vi "non_linear_fitting_multiple.vi"(11 "Graph array":cluster{"output":dbl[], "output":dbl[]}[](array[cluster])=[{"output"=array[10000 elements], "output"=array[10000 elements]}]) -> (0 "error out":errorcluster)   [LabVIEW 2025]
panel:
  in  "Old Fitting functions":string="standard streched expnental + power decay\n: (a0+a1*x^(a2)*exp(-(x/a3)^a4)\nstreched exponential with modified constants for x=0,limitless\n:(a0-a1)*exp(-(x/a2)^a3)+a1"
  out "Numeric":i32
  in  "fitting param col.":i32
  out "fitting parameter plot":cluster{dbl[], dbl[]}(graph)
  out "best fit parameter":dbl[](array[numeric])
  in  "Fitting Function":string="(a0-a1)*exp(-(x/a2)^a3)+a1"
  in  "Parameter array":T1(array[cluster])=[{"initial param"=0.0, "variable?"=TRUE, "lower limit"=0.0, "upper limit"=0.0, "name"="a0"}, {"initial param"=0.0, "variable?"=TRUE, "lower limit"=0.0, "upper limit"=0.0, "name"="a1"}, {"initial param"=0.0, "variable?"=FALSE, "lower limit"=0.0, "upper limit"=0.0, "name"="a2"}, {"initial param"=0.0, "variable?"=TRUE, "lower limit"=0.0, "upper limit"=0.0, "name"="a3"}, {"initial param"=0.0, "variable?"=TRUE, "lower limit"=0.0, "upper limit"=0.0, "name"="a4"}]
  in  "?":cluster{"max iteration":i32, "tolerance":dbl}={"max iteration"=100000, "tolerance"=1e-20}
  out "spreadsheet string 2":string
  out "spreadsheet string":string
  in  "OK Button":bool
  out "raw data":cluster{"output":dbl[], "output":dbl[]}(graph)
  in  "use variables":bool
  out "Fitting":T2(graph)
  in  "variable":string="4.2\n3.5"
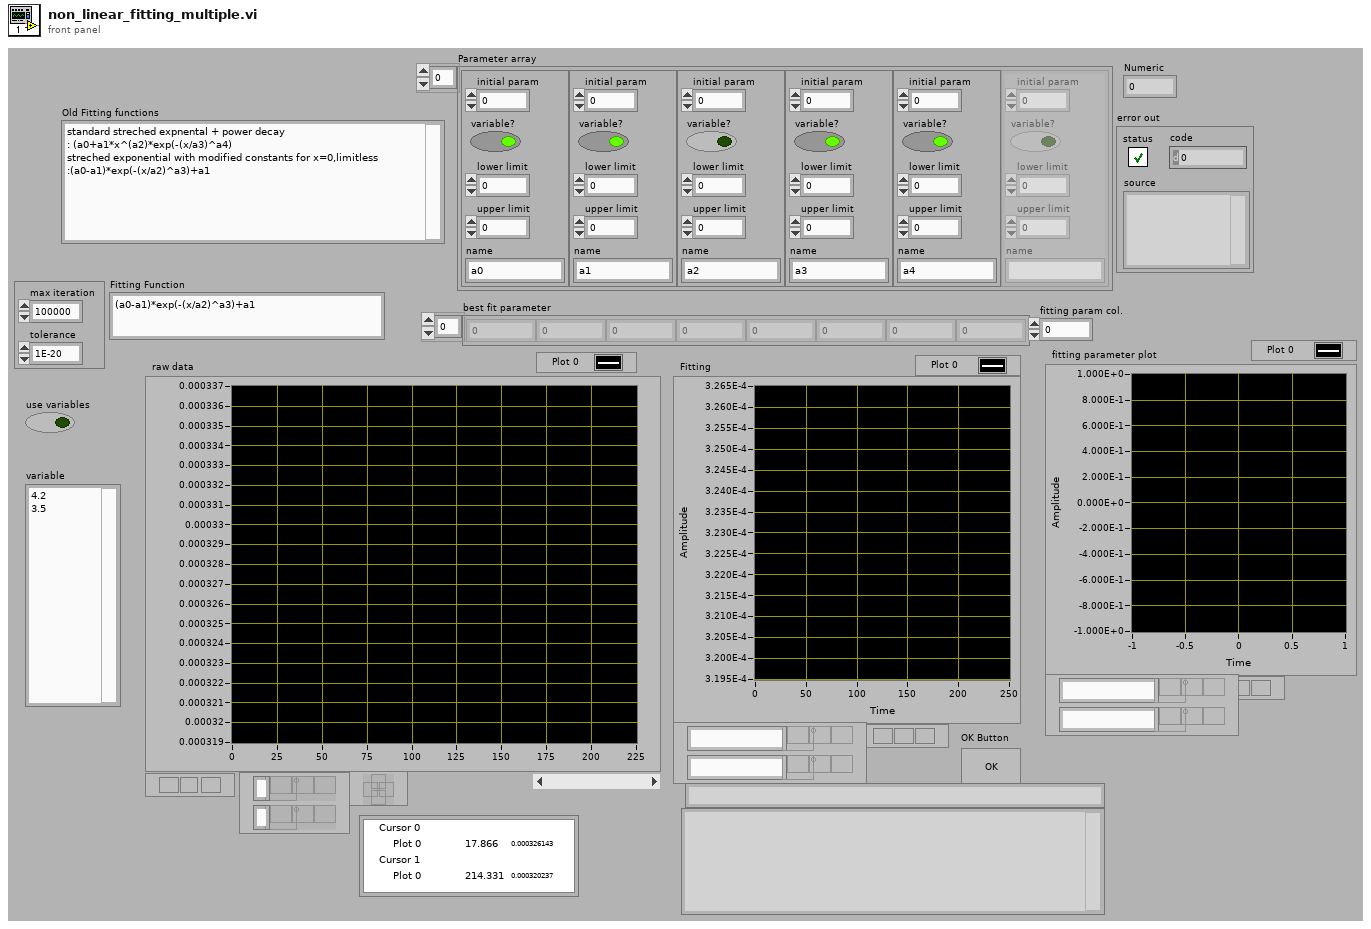
[diagram p1: front panel]
types:
  T1 = cluster{"initial param":dbl, "variable?":bool, "lower limit":dbl, "upper limit":dbl, "name":string}[]
  T2 = cluster{"array out":dbl[], "Best Exponential Fit":dbl[]}[]
  T3 = typedef "LVCursorListTypeDef.ctl" = cluster{"Name":string, "Color":u32, "Style":u8, "Point Style":u8, "Name Visible":bool, "Allow Drag":bool, "Cursor Mode":u32, "Plot":i32, "Index":i32, "Position":cluster{"X":dbl, "Y":dbl}, "X Scale":u32, "Y Scale":u32, "Watch Plots":i32[], "Watch All Plots":bool, "Plot Area":i32, "Label Offset":cluster{"X":dbl, "Y":dbl}}[]
  T4 = cluster{"array out":dbl[], "best nonlinear fit":dbl[]}
  T5 = cluster{"array out":dbl[], "best nonlinear fit":dbl[]}[]
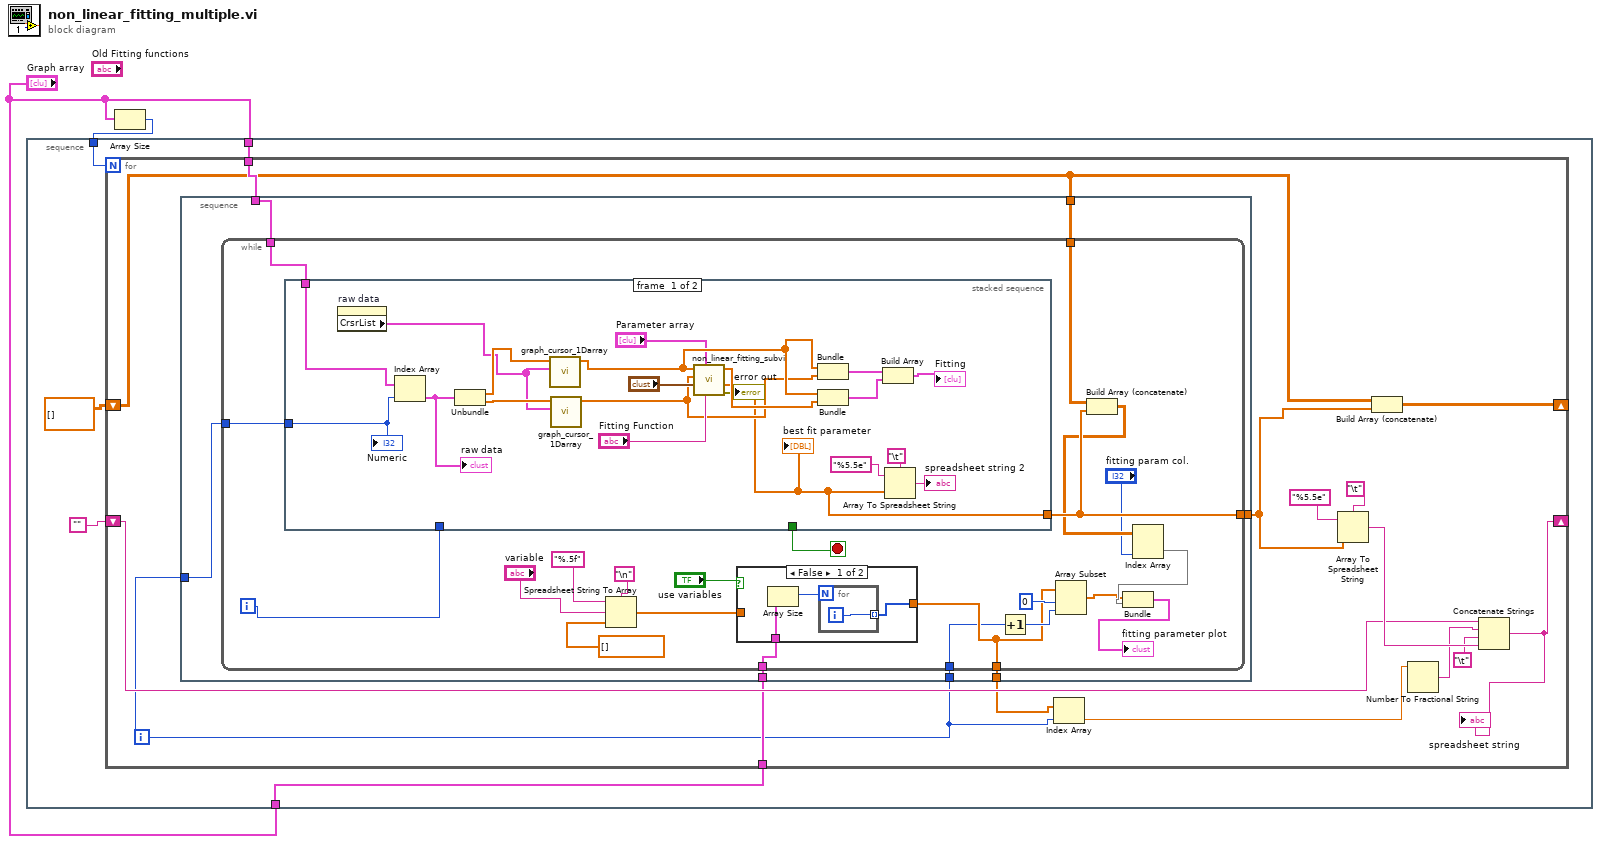
[diagram p0: block diagram]
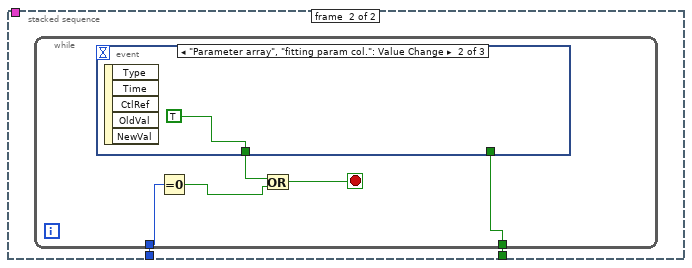
[diagram p3: hidden frame]
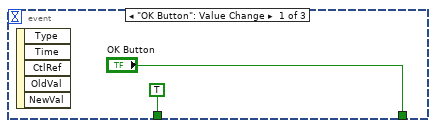
[diagram p4: hidden frame]
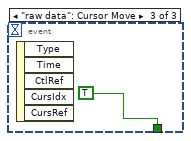
[diagram p5: hidden frame]
diagram:
  n1 = Array Size(array="Graph array") -> (size(s)=w2:i32)
  n2 = stacked-sequence {
    tunnel: "Graph array" -> [w7]
    tunnel: "Graph array" -> [w3]
    tunnel: w2 -> [w4]
    frame #0 {
      n3 = for {
        N: w4 -> [_]
        tunnel: w7 -> [w22]
        shift-right: [w17] -> _
        shift-left: dbl[][] [] -> [w11]
        shift-right: [w20] -> _
        shift-left: "" -> [w15]
        tunnel: w3 -> [w12]
        i -> [w9]
        n4 = stacked-sequence {
          tunnel: w22 -> [w29]
          tunnel: w9 -> [w27]
          tunnel: [w28] -> w18
          tunnel: w12 -> [w26]
          tunnel: [w25] -> w10
          tunnel: w9 -> [w24]
          tunnel: w11 -> [w23]
          frame #0 {
            n5 = while {
              tunnel: w29 -> [w51]
              tunnel: [w32] -> w28
              tunnel: w27 -> [w48]
              tunnel: w26 -> [w34]
              tunnel: [w39] -> w25
              tunnel: w24 -> [w35]
              tunnel: w23 -> [w33]
              i -> [w50]
              stop <- w49 stop-if-true
              n6 = stacked-sequence {
                tunnel: w51 -> [w76 _]
                tunnel: w50 -> [_ w78]
                tunnel: [_ w77] -> w49
                tunnel: [w60 _] -> w32
                tunnel: w48 -> [w58 _]
                frame #0 {
                  n7 = property on="raw data" class="XYGraph (strict)"() -> ("CrsrList"=w70:T3)  [unwired: 2 in, 2 out]
                  n8 = Index Array(array=w76, index=w58) -> (element=w57:cluster{"output":dbl[], "output":dbl[]})
                  "raw data" <- w57
                  n9 = Unbundle(w57) -> ("output"=w75:dbl[], "output"=w74:dbl[])
                  n10 = call "graph_cursor_1Darray.vi"("Cusor list"=w70, "array in"=w75) -> ("array out"=w64:dbl[])  [unwired: 9 in]
                  n11 = call "graph_cursor_1Darray.vi"("Cusor list"=w70, "array in"=w74) -> ("array out"=w61:dbl[])  [unwired: 9 in]
                  n12 = call "non_linear_fitting_subvi.vi"("Fitting Function"="Fitting Function", "Parameter array"="Parameter array", "termination"="?", "Y"=w61, "X"=w64) -> ("error out"=→"error out":errorcluster, "best fit parameter"=w60:dbl[], "best nonlinear fit"=w65:dbl[])  [unwired: 3 in, 1 out]
                  "best fit parameter" <- w60
                  n13 = Bundle("array out"=w64, "array out"=w61) -> (w73:cluster{"array out":dbl[], "array out":dbl[]})  [unwired: 1 in]
                  n14 = Bundle("array out"=w64, "best nonlinear fit"=w65) -> (w72:T4)  [unwired: 1 in]
                  n15 = Build Array(w73, w72) -> (→"Fitting":T5)
                  n16 = Array To Spreadsheet String(delimiter (Tab)="\t", array=w60, 3:"%5.5e" ("format string")) -> (spreadsheet string=→"spreadsheet string 2":string)
                  "Numeric" <- w58
                }
                frame #1 {
                  n17 = while {
                    tunnel: w78 -> [w82]
                    tunnel: [w80] -> w77
                    stop <- w81 stop-if-true
                    n18 = event shown="[1] \"Parameter array\", \"fitting param col.\": Value Change" {
                      selector: _ -> [_ _ _]
                      dyn-events: _ -> [_ _ _]
                      timeout: _ -> [_ _ _]
                      tunnel: [TRUE ("OK Button 2") TRUE ("OK Button 2") TRUE ("OK Button 2")] -> w83
                      tunnel: ["OK Button" _ _] -> w80
                      event "OK Button": Value Change {
                        n19 = event-data() -> ()  [unwired: 1 in, 5 out]
                      }
                      event "Parameter array", "fitting param col.": Value Change {
                        n20 = event-data() -> ()  [unwired: 1 in, 5 out]
                      }
                      event "raw data": Cursor Move {
                        n21 = event-data() -> ()  [unwired: 1 in, 5 out]
                      }
                    }
                    n22 = Equal To 0?(x=w82) -> (x = 0?=w79:bool)
                    n23 = Or(x=w83, y=w79) -> (x .or. y?=w81:bool)
                  }
                }
              }
              n24 = Spreadsheet String To Array(delimiter (Tab)="\n", format string="%.5f", spreadsheet string="variable", array type (2D Dbl)=dbl[] []) -> (array=w47:dbl[])
              n25 = case shown="False" "use variables" {
                tunnel: w47 -> [_ w56]
                tunnel: [w53 w56] -> w39
                tunnel: w34 -> [w52 _]
                frame False {
                  n26 = Array Size(array=w52) -> (size(s)=w54:i32)
                  n27 = for {
                    N: w54 -> [_]
                    tunnel: [w55] -> w53 mode=indexing
                    i -> [w55]
                  }
                }
                frame True {
                }
              }
              n28 = Increment(x=w35) -> (x+1=w40:i32)
              n29 = Array Subset(array=w39, index=0, length=w40) -> (w37:dbl[])
              n30 = Build Array (concatenate)(w33, w32) -> (w31:dbl[][])
              n31 = Index Array(array=w31, index (col)="fitting param col.") -> (element=w38:dbl[])  [unwired: 1 in]
              n32 = Bundle(w37, w38) -> (→"fitting parameter plot":cluster{dbl[], dbl[]})  [unwired: 1 in]
            }
          }
        }
        n33 = Index Array(array=w10, index=w9) -> (element=w8:dbl)
        n34 = Array To Spreadsheet String(delimiter (Tab)="\t", array=w18, 3:"%5.5e" ("format string")) -> (spreadsheet string=w19:string)
        n35 = Build Array (concatenate)(w11, w18) -> (w17:dbl[][])
        n36 = Number To Fractional String(number=w8) -> (F-format string=w14:string)  [unwired: 3 in]
        n37 = Concatenate Strings(w15, w14, "\t", w19) -> (w20:string)
        "spreadsheet string" <- w20
      }
    }
  }
